vi "SENS_SWE_TRIG_DEL.vi"(0 "VISA IN":refnum<visa-resource-name>, 1 "Trigger Delay(sec)":i32, 5 "error in":errorcluster, 7 "Channel":i32) -> (14 "VISA Out":refnum<visa-resource-name>, 19 "error out":errorcluster)   [LabVIEW 2018, in "PNA-X.lvlib"]
doc: "SENSe<cnum>:SWEep:TRIGger:DELay <num> \n(Read-Write) Sets and reads the trigger delay for all measurements in the specified CHANNEL. This delay is only \napplied while TRIG:SOURce EXTernal and TRIG:SCOP CURRent . After an external trigger is applied, the start \nof the sweep is delayed for the specified delay value plus any inherent latency. \nTo apply a trigger delay for all channels (Global), use TRIG:DEL \nParameters \n<cnum> Any existing channel number. If unspecified, value is set to 1 \n<num> Trigger delay value in seconds. Range is from 0 to 107 seconds \nExamples SENS:SWE:TRIG:DELay .003 \nsense2:sweep:trigger:delay 1 \nQuery Syntax SENSe<cnum>:SWEep:TRIGger:DELay? \nReturn Type Numeric \nDefault 0"
uses:
  PNA-X.lvlib
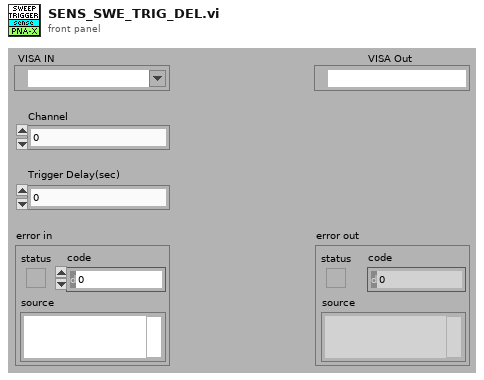
[diagram p1: front panel]
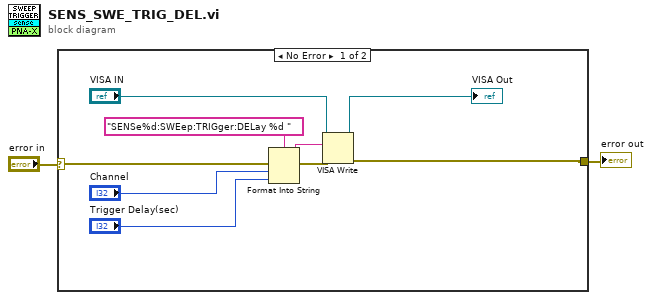
[diagram p0: block diagram]
diagram:
  n1 = case shown="No Error" "error in" {
    selector: "error in" -> [w11 w12]
    tunnel: [w6 w12] -> w1
    frame No Error {
      n2 = Format Into String(format string="SENSe%d:SWEep:TRIGger:DELay %d " ("Cmdline"), error in=w11, "Channel", "Trigger Delay(sec)") -> (resulting string=w9:string, error out=w10:errorcluster)  [unwired: 1 in]
      n3 = VISA Write(VISA resource name="VISA IN", write buffer=w9, error in (no error)=w10) -> (VISA resource name out=→"VISA Out":refnum<visa-resource-name>, error out=w6:errorcluster)  [unwired: 1 out]
    }
    frame Error {
    }
  }
  "error out" <- w1
